vi "Read_Arduino_Variant.vi"(8 "error in (no error)":errorcluster, 9 "Variant":variant) -> (0 "error out":errorcluster, 2 "Channels":u8)   [LabVIEW 2023]
uses:
  <userlib>/_OpenG.lib/lvdata/lvdata.llb/openg_variant.lvlib
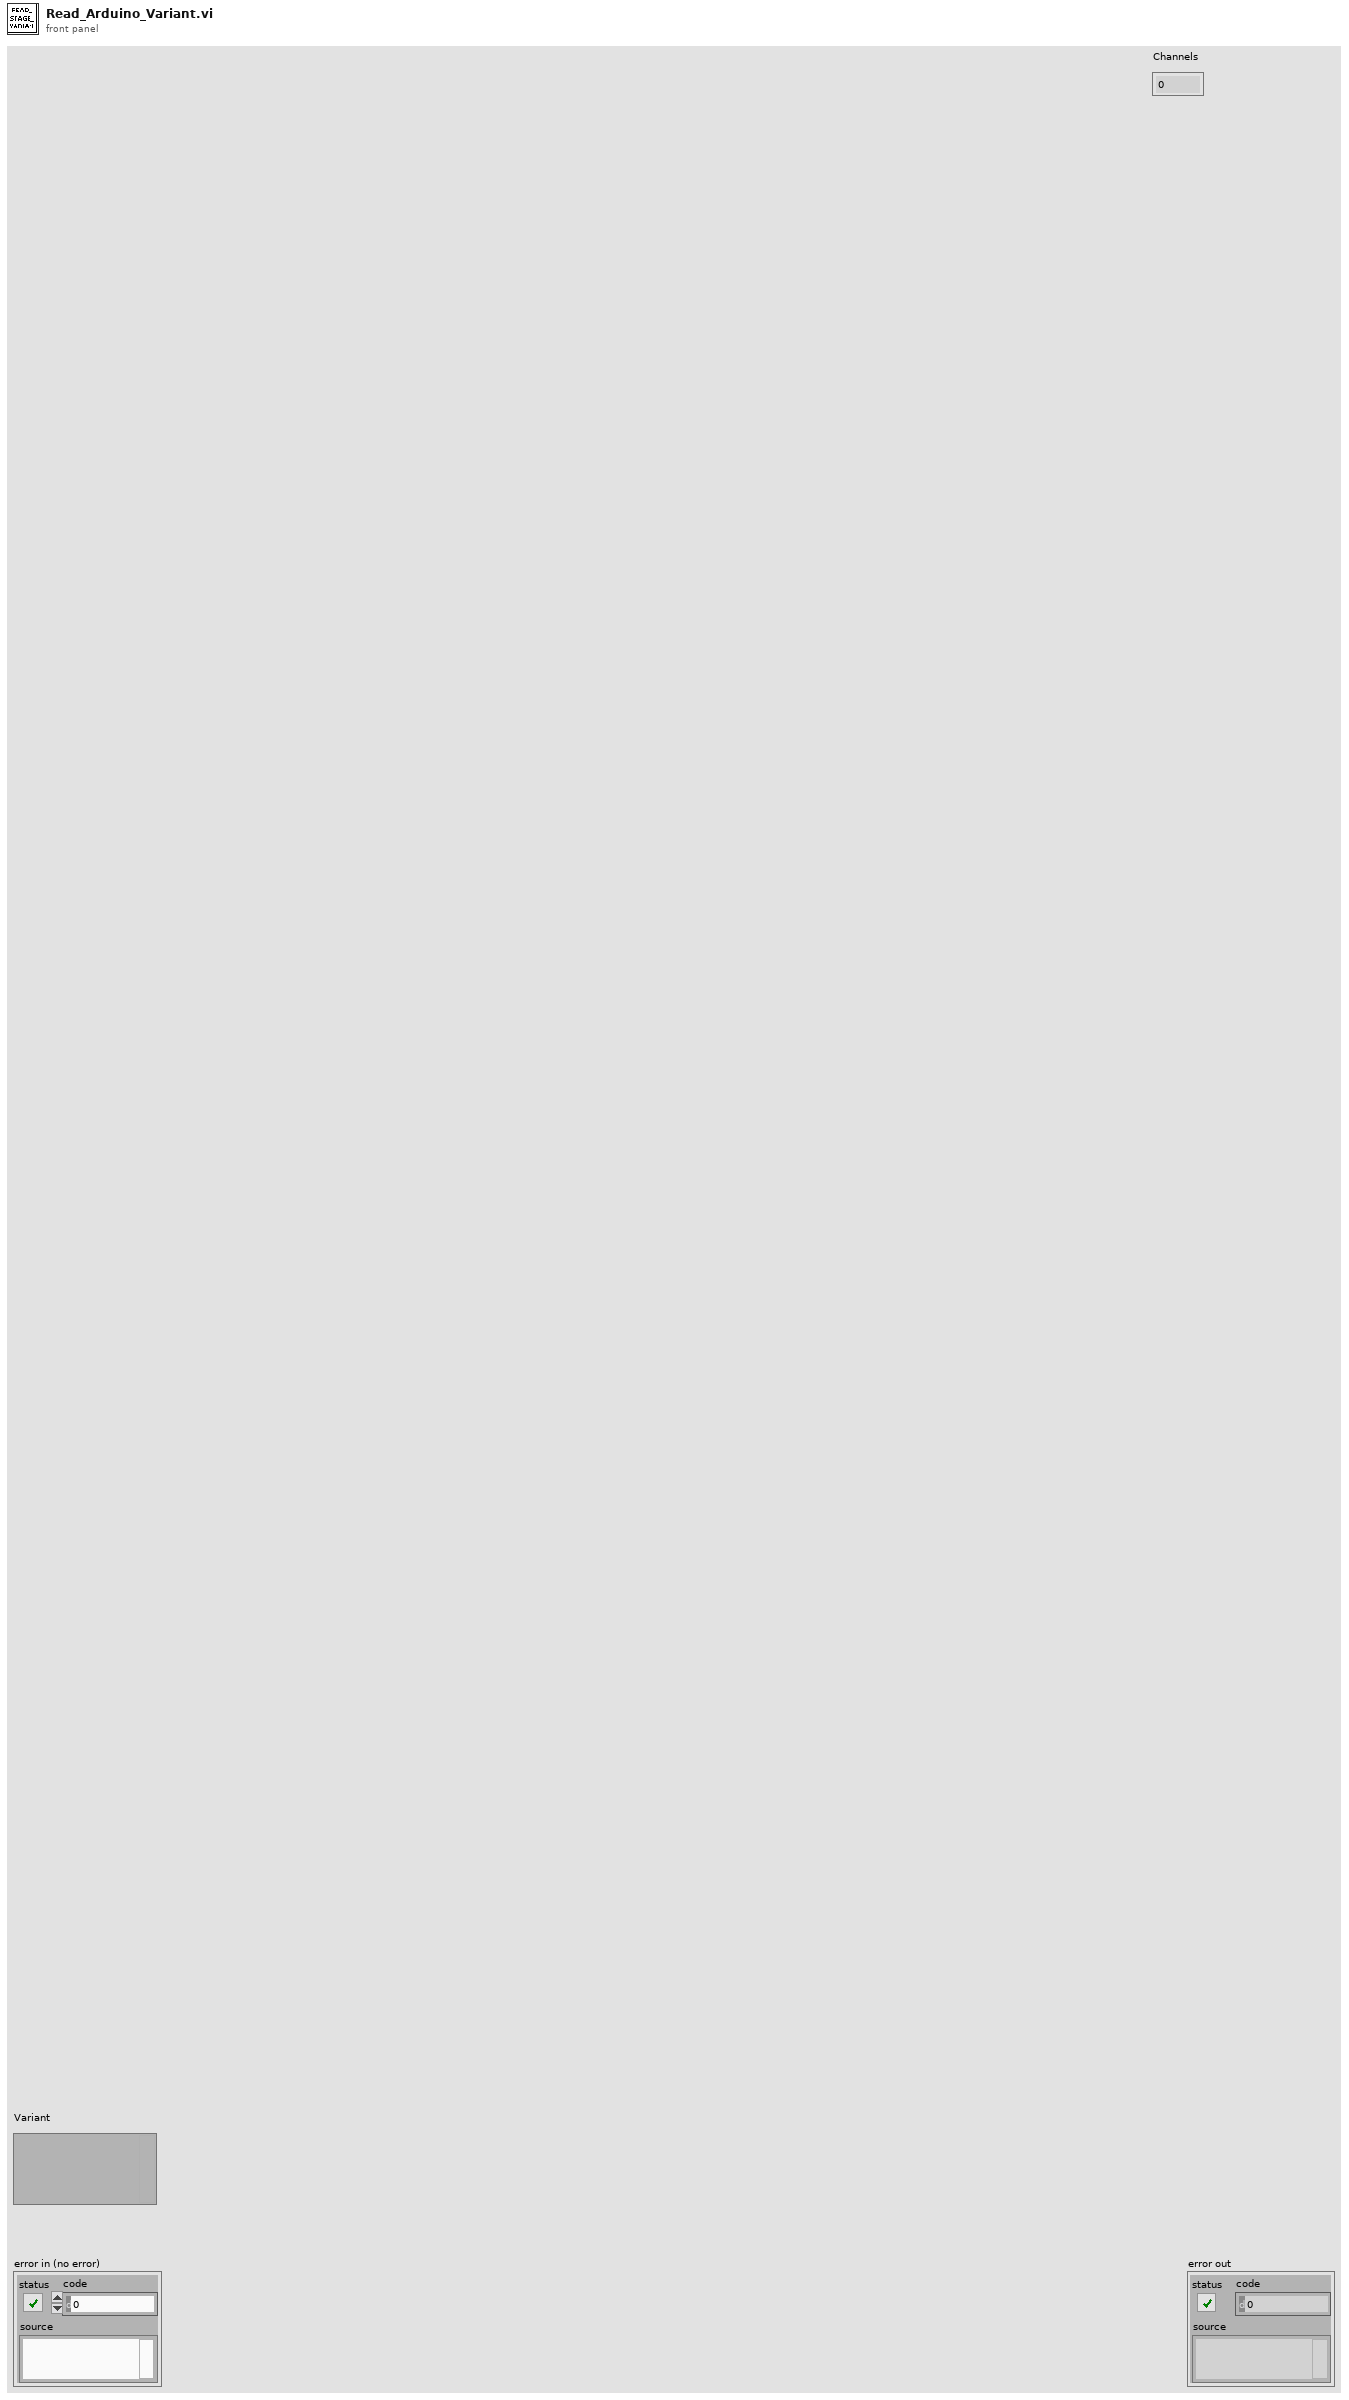
[diagram p1: front panel]
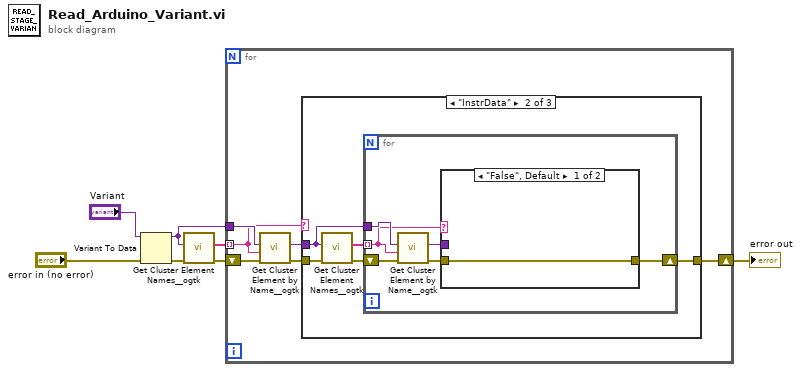
[diagram p0: block diagram]
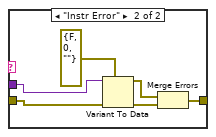
[diagram p3: hidden frame]
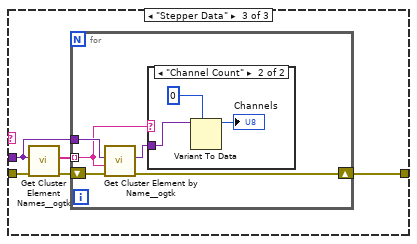
[diagram p4: hidden frame]
diagram:
  n1 = Variant To Data(error in="error in (no error)", Variant="Variant") -> (data=w4:variant, error out=w6:errorcluster)  [unwired: 1 in]
  n2 = call <userlib>:"Get Cluster Element Names__ogtk.vi"("error in (no error)"=w6, "Cluster"=w4) -> ("error out"=w5:errorcluster, "Element Names"=w3:string[])  [unwired: 8 in]
  n3 = for {
    tunnel: w3 -> [w12] mode=indexing
    tunnel: w4 -> [w13]
    shift-right: [w8] -> w7
    shift-left: w5 -> [w9]
    n4 = call <userlib>:"Get Cluster Element by Name__ogtk.vi"("error in (no error)"=w9, "Element Name"=w12, "Cluster"=w13) -> ("error out"=w10:errorcluster, "VElement"=w11:variant)  [unwired: 6 in, 1 out]
    n5 = case shown="\"InstrData\"" w12 {
      tunnel: w11 -> [_ w18 w36]
      tunnel: w10 -> [w14 w17 w35]
      tunnel: [w14 w15 w33] -> w8
      frame "False", Default {
      }
      frame "InstrData" {
        n6 = call <userlib>:"Get Cluster Element Names__ogtk.vi"("error in (no error)"=w17, "Cluster"=w18) -> ("error out"=w16:errorcluster, "Element Names"=w19:string[])  [unwired: 8 in]
        n7 = for {
          tunnel: w19 -> [w24] mode=indexing
          tunnel: w18 -> [w25]
          shift-right: [w20] -> w15
          shift-left: w16 -> [w22]
          n8 = call <userlib>:"Get Cluster Element by Name__ogtk.vi"("error in (no error)"=w22, "Element Name"=w24, "Cluster"=w25) -> ("error out"=w21:errorcluster, "VElement"=w23:variant)  [unwired: 6 in, 1 out]
          n9 = case shown="\"False\", Default" w24 {
            tunnel: w23 -> [_ w32]
            tunnel: w21 -> [w26 w30]
            tunnel: [w26 w27] -> w20
            frame "False", Default {
            }
            frame "Instr Error" {
              n10 = Variant To Data(error in=w30, type=errorcluster {"status"=FALSE, "code"=0, "source"=""} ("error out"), Variant=w32) -> (data=w29:errorcluster, error out=w28:errorcluster)
              n11 = Merge Errors(w29, w28) -> (w27:errorcluster)
            }
          }
        }
      }
      frame "Stepper Data" {
        n12 = call <userlib>:"Get Cluster Element Names__ogtk.vi"("error in (no error)"=w35, "Cluster"=w36) -> ("error out"=w34:errorcluster, "Element Names"=w37:string[])  [unwired: 8 in]
        n13 = for {
          tunnel: w37 -> [w41] mode=indexing
          tunnel: w36 -> [w42]
          shift-right: [w38] -> w33
          shift-left: w34 -> [w39]
          n14 = call <userlib>:"Get Cluster Element by Name__ogtk.vi"("error in (no error)"=w39, "Element Name"=w41, "Cluster"=w42) -> ("error out"=w38:errorcluster, "VElement"=w40:variant)  [unwired: 6 in, 1 out]
          n15 = case shown="\"Channel Count\"" w41 {
            tunnel: w40 -> [_ w45]
            frame "False", Default {
            }
            frame "Channel Count" {
              n16 = Variant To Data(type=u8 0, Variant=w45) -> (data=→"Channels":u8)  [unwired: 1 in, 1 out]
            }
          }
        }
      }
    }
  }
  "error out" <- w7
